vi "MainControlGUI.vi"() -> ()   [LabVIEW 2016]
uses:
  <vilib>/Platform/TimedLoop/XDataNode/timing_clust.ctl
  <vilib>/Platform/TimedLoop/XDataNode/nitl_modes.ctl
  <vilib>/Platform/TimedLoop/XDataNode/wakeup.ctl
  S2017_ControlCode/src/mainControl/podGlobals_9066.vi
  <vilib>/platform/TimedLoop/XDataNode/XDataNode.xnode
  <vilib>/Platform/TimedLoop/XDataNode/XDNodeRunTimeDep.lvlib
panel:
  in  "LM335Z Raw (V)":dbl
  out "LM335Z Temp (C)":dbl format="%#_13g"
  in  "MCP9700 Raw (V)":dbl
  out "MCP9700 Temp (C)":dbl format="%#_13g"
  in  "Update Rate (ms)":dbl=1.0 min=10.0
  in  "STOP":bool
  in  "TMP36 Raw (V)":dbl
  out "TMP36 Temp (C)":dbl format="%#_13g"
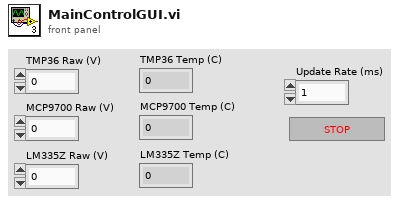
[diagram p1: front panel]
types:
  T1 = typedef "XDNodeRunTimeDep.lvlib/timing_clust.ctl" = cluster{"Expected End [f-1]":u64, "Actual End [f-1]":u64, "Finished Late? [f-1]":bool, "Expected End [i-1]":u64, "Actual End [i-1]":u64, "Finished Late? [i-1]":bool, "Expected Start [i]":u64, "Actual Start [i]":u64, "Expected Start [f]":u64, "Actual Start [f]":u64, "Source Name":string, "Structure Name":string, "Period":i64, "Deadline":i64, "Offset":i64, "Start":i64, "Priority":i32, "Timeout":i32, "Mode":T2, "Wakeup Reason":T3, "Error":errorcluster, "Source Type":string, "Secondary Source Type":string, "Global End Time":u64, "Global Start Time":u64, "Frame Duration":u64, "Iteration Duration":u64, "Assigned CPU":i32, "I/O Scan Engine Mode":u32}
  T2 = typedef "XDNodeRunTimeDep.lvlib/nitl_modes.ctl" = enum32{"No Change", "Process missed periods, maintain original phase", "Discard missed periods, maintain original phase", "Process missed periods, ignore original phase", "Discard missed periods, ignore original phase"}
  T3 = typedef "XDNodeRunTimeDep.lvlib/wakeup.ctl" = enum32{"Normal", "Aborted", "Asynchronous wakeup", "Timing source error", "Timed loop error", "Timeout"}
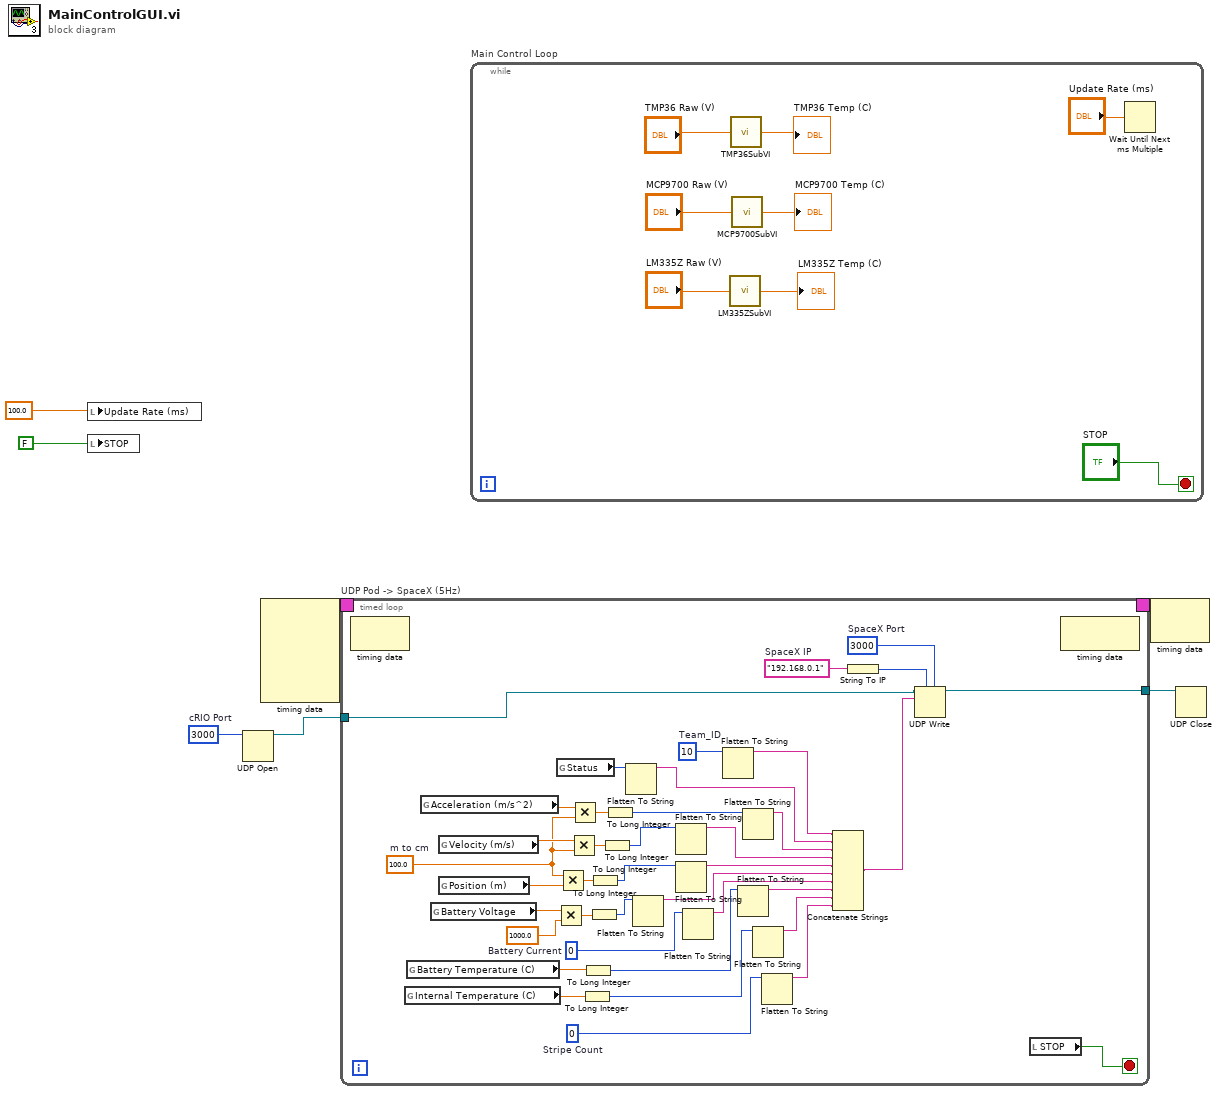
[diagram p0: block diagram]
diagram:
  w5 = u32 3000  # cRIO Port
  n1 = local write "Update Rate (ms)"(100.0) -> ()
  n2 = local write "STOP"(FALSE) -> ()
  n3 = UDP Open(11:w5) -> (port=w4:refnum<k16>)  [unwired: 4 in, 2 out]
  n4 = node-c288() -> (w7:T1)  [unwired: 5 in]
  n5 = timed-loop "UDP Pod -> SpaceX (5Hz)" {
    timing: w7 -> [_]
    timing-out: [_] -> w6
    tunnel: w4 -> [w10]
    tunnel: [w9] -> w3
    stop <- w8 stop-if-true
    w11 = u32 0  # Stripe Count
    w17 = 0  # Battery Current
    w43 = 100.0  # m to cm
    w29 = u8 10  # Team_ID
    w31 = u16 3000  # SpaceX Port
    w34 = "192.168.0.1"  # SpaceX IP
    n6 = node-c288() -> ()  [unwired: 1 in, 1 out]
    n7 = global read "podGlobals_9066.vi" "Internal Temperature (C)"() -> (w35:dbl)
    n8 = global read "podGlobals_9066.vi" "Battery Temperature (C)"() -> (w36:dbl)
    n9 = global read "podGlobals_9066.vi" "Acceleration (m/s^2)"() -> (w46:dbl)
    n10 = global read "podGlobals_9066.vi" "Battery Voltage"() -> (w37:dbl)
    n11 = global read "podGlobals_9066.vi" "Velocity (m/s)"() -> (w45:dbl)
    n12 = global read "podGlobals_9066.vi" "Position (m)"() -> (w44:dbl)
    n13 = Multiply(x=w37, y=1000.0) -> (x*y=w39:dbl)
    n14 = global read "podGlobals_9066.vi" "Status"() -> (w27:u8)
    n15 = Multiply(x=w43, y=w44) -> (x*y=w40:dbl)
    n16 = Multiply(x=w45, y=w43) -> (x*y=w41:dbl)
    n17 = Multiply(x=w46, y=w43) -> (x*y=w42:dbl)
    n18 = To Long Integer(number=w35) -> (32bit integer=w13:i32)
    n19 = To Long Integer(number=w36) -> (32bit integer=w15:i32)
    n20 = To Long Integer(number=w39) -> (32bit integer=w19:i32)
    n21 = To Long Integer(number=w40) -> (32bit integer=w21:i32)
    n22 = To Long Integer(number=w41) -> (32bit integer=w23:i32)
    n23 = To Long Integer(number=w42) -> (32bit integer=w26:i32)
    n24 = Flatten To String(anything=w27) -> (data string=w28:string)  [unwired: 3 in, 2 out]
    n25 = Flatten To String(anything=w19) -> (data string=w20:string)  [unwired: 3 in, 2 out]
    n26 = Flatten To String(anything=w23) -> (data string=w24:string)  [unwired: 3 in, 2 out]
    n27 = Flatten To String(anything=w21) -> (data string=w22:string)  [unwired: 3 in, 2 out]
    n28 = Flatten To String(anything=w17) -> (data string=w18:string)  [unwired: 3 in, 2 out]
    n29 = Flatten To String(anything=w29) -> (data string=w30:string)  [unwired: 3 in, 2 out]
    n30 = Flatten To String(anything=w15) -> (data string=w16:string)  [unwired: 3 in, 2 out]
    n31 = Flatten To String(anything=w26) -> (data string=w25:string)  [unwired: 3 in, 2 out]
    n32 = Flatten To String(anything=w13) -> (data string=w14:string)  [unwired: 3 in, 2 out]
    n33 = Flatten To String(anything=w11) -> (data string=w12:string)  [unwired: 3 in, 2 out]
    n34 = Concatenate Strings(w30, w28, w25, w24, w22, w20, w18, w16, w14, w12) -> (w33:string)
    n35 = String To IP(1:w34) -> (0:w32:u32)
    n36 = UDP Write(address=w32, port or service name=w31, connection ID=w10, data in=w33) -> (3:w9:refnum<k16>)  [unwired: 2 in, 1 out]
    n37 = local read "STOP"() -> (w8:bool)
    n38 = node-c288() -> ()  [unwired: 1 in, 1 out]
  }
  n39 = while "Main Control Loop" {
    stop <- "STOP" stop-if-true
    n40 = call "LM335ZSubVI.vi"("Raw Input (V)"="LM335Z Raw (V)") -> ("Temperature (C)"=→"LM335Z Temp (C)":dbl)
    n41 = call "TMP36SubVI.vi"("Raw Input (V)"="TMP36 Raw (V)") -> ("Temperature (C)"=→"TMP36 Temp (C)":dbl)
    n42 = call "MCP9700SubVI.vi"("Raw Input (V)"="MCP9700 Raw (V)") -> ("Temperature (C)"=→"MCP9700 Temp (C)":dbl)
    n43 = Wait Until Next ms Multiple(millisecond multiple="Update Rate (ms)") -> ()  [unwired: 1 out]
  }
  n44 = node-c288(w6) -> ()  [unwired: 1 out]
  n45 = UDP Close(connection ID=w3) -> ()  [unwired: 1 in, 2 out]
